vi "process.vi"(8 "error in":errorcluster, 9 "result allocation":T1, 10 "parameters":T1, 11 "module in":refnum<class "fixed channel tag bus module.lvclass">) -> (0 "error out":errorcluster, 1 "results":T1, 2 "parameter allocation":T1, 3 "module out":refnum<class "fixed channel tag bus module.lvclass">)   [LabVIEW 2013, in "fixed channel tag bus module.lvclass"]
doc: "Provides an interface for information processing by a module at runtime. While this interface performs no operations, a child should provide an override which may process data in any manner necessary."
uses:
  fixed channel tag bus module.lvclass
  <vilib>/NI/Tag Bus/table/data table.ctl
  fixed channel tag bus module.lvclass/fixed channel tag bus module.ctl
  <vilib>/NI/Tag Bus/table/data polymorphs/read one/read Double.vi
  <vilib>/NI/Tag Bus/table/data polymorphs/write one/write Double.vi
  <vilib>/NI/Tag Bus/table/data table.lvlib
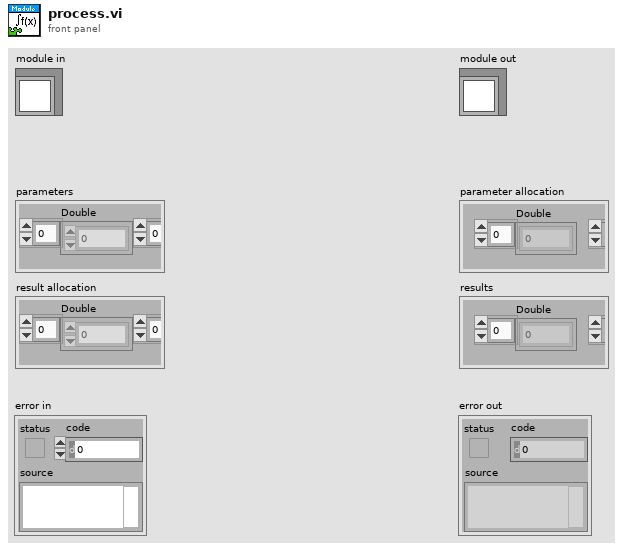
[diagram p1: front panel]
types:
  T1 = typedef "tag bus.lvlib/data table.lvlib/data table.ctl" = cluster{"Double":dbl[], "Single":sgl[], "I64":i64[], "I32":i32[], "I16":i16[], "I8":i8[], "U64":u64[], "U32":u32[], "U16":u16[], "U8":u8[], "Boolean":bool[], "String":string[], "Array of Double":cluster{"DBL Array":dbl[]}[], "Array of Single":cluster{"SGL Array":sgl[]}[], "Array of I64":cluster{"I64 Array":i64[]}[], "Array of I32":cluster{"I32 Array":i32[]}[], "Array of I16":cluster{"I16 Array":i16[]}[], "Array of I8":cluster{"I8 Array":i8[]}[], "Array of U64":cluster{"U64 Array":u64[]}[], "Array of U32":cluster{"U32 Array":u32[]}[], "Array of U16":cluster{"U16 Array":u16[]}[], "Array of U8":cluster{"U8 Array":u8[]}[], "Array of Boolean":cluster{"Boolean Array":bool[]}[], "Array of String":cluster{"String Array":string[]}[]}
  T2 = typedef "fixed channel tag bus module.lvclass/parameters.ctl" = cluster{"placeholder":i32}
  T3 = typedef "fixed channel tag bus module.lvclass/results.ctl" = cluster{"placeholder":i32}
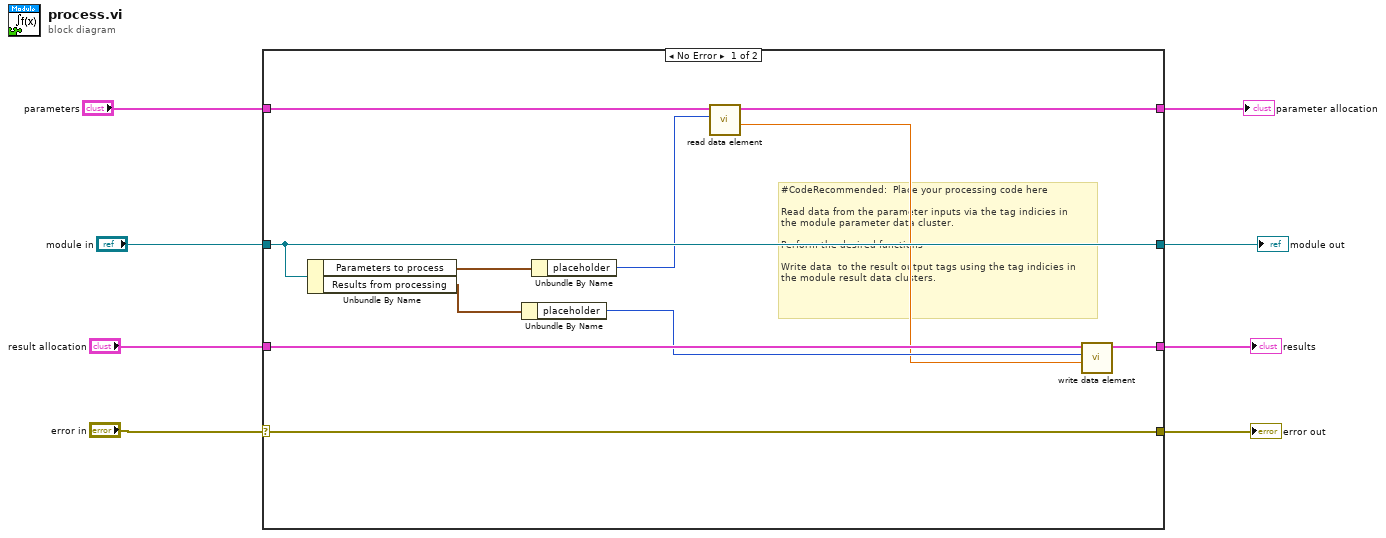
[diagram p0: block diagram]
diagram:
  n1 = case shown="No Error" "error in" {
    selector: "error in" -> [w19 w20]
    tunnel: [w19 w20] -> w7
    tunnel: "module in" -> [w18 w23]
    tunnel: "parameters" -> [w15 w22]
    tunnel: [w14 w22] -> w4
    tunnel: "result allocation" -> [w13 w21]
    tunnel: [w12 w21] -> w2
    tunnel: [w18 w23] -> w1
    frame No Error {
      # "#CodeRecommended:  Place your processing code here\n\nRead data from the parameter inputs via the tag indicies in\nthe module parameter data cluster.\n\nPerform the desired functions\n\nWrite data  to the result output tags using the tag indicies in\nthe module result data clusters."
      n2 = Unbundle By Name(w18) -> ("Parameters to process"=w17:T2, "Results from processing"=w16:T3)
      n3 = Unbundle By Name(w16) -> ("placeholder"=w10:i32)
      n4 = Unbundle By Name(w17) -> ("placeholder"=w11:i32)
      n5 = call-poly <vilib>:"read data element.vi"("index"=w11, "data table in"=w15) -> ("value"=w9:dbl, "data table out"=w14:T1)  [unwired: 8 in]
      n6 = call-poly <vilib>:"write data element.vi"("value"=w9, "index"=w10, "data table in"=w13) -> ("data table out"=w12:T1)  [unwired: 8 in]
    }
    frame Error {
    }
  }
  "error out" <- w7
  "module out" <- w1
  "results" <- w2
  "parameter allocation" <- w4
